vi "Caraya Test for Find Complete Frame.vi"() -> ()   [LabVIEW 2018]
uses:
  Libraries/iTacho_class/iTacho.lvclass
  <vilib>/addons/_JKI Toolkits/Caraya/classes/Test/Test.lvclass
  <vilib>/addons/_JKI Toolkits/Caraya/classes/Assert/Assert.lvclass
panel:
  out "error out":errorcluster
  out "Test Pass?":bool
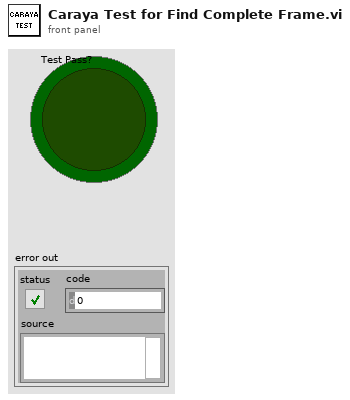
[diagram p1: front panel]
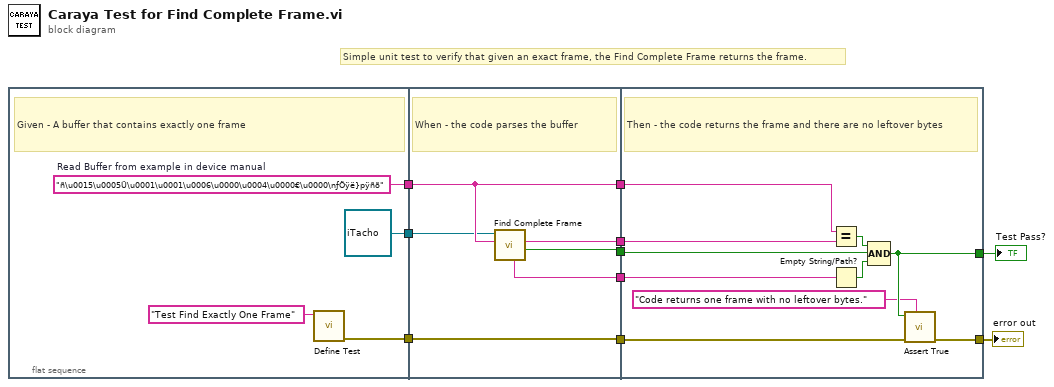
[diagram p0: block diagram]
diagram:
  # "Simple unit test to verify that given an exact frame, the Find Complete Frame returns the frame."
  n1 = flat-sequence {
    tunnel: [refnum<class "iTacho.lvclass"> refnum ("iTacho in")] -> w10
    tunnel: [w13] -> w9
    tunnel: [w11] -> w2
    tunnel: w10 -> [w19]
    tunnel: w9 -> [w20]
    tunnel: [w20] -> w8
    tunnel: [w18] -> w7
    tunnel: [w17] -> w6
    tunnel: [w16] -> w5
    tunnel: [w15] -> w3
    tunnel: w2 -> [w15]
    tunnel: w8 -> [w25]
    tunnel: w7 -> [w28]
    tunnel: w6 -> [w26]
    tunnel: w5 -> [w27]
    tunnel: [w23] -> w4
    tunnel: w3 -> [w24]
    tunnel: [w21] -> w1
    frame #0 {
      w13 = "ñ\u0015\u0005Ü\u0001\u0001\u0006\u0000\u0004\u0000€\u0000\nƒÖÿë}pÿñõ"  # Read Buffer from example in device manual
      # "Given - A buffer that contains exactly one frame"
      n2 = call <vilib>:"Define Test.vi"("Label (VI Title)"="Test Find Exactly One Frame") -> ("error out"=w11:errorcluster)  [unwired: 10 in]
    }
    frame #1 {
      # "When - the code parses the buffer"
      n3 = call-dynamic "Find Complete Frame.vi"("Read Buffer in"=w20, "iTacho in"=w19) -> ("Found New Frame?"=w18:bool, "Frame"=w17:string, "Leftover Bytes"=w16:string)  [unwired: 5 in, 2 out]
    }
    frame #2 {
      # "Then - the code returns the frame and there are no leftover bytes"
      n4 = Equal?(x=w25, y=w26) -> (x = y?=w29:bool)
      n5 = Empty String/Path?(string/path=w27) -> (empty?=w30:bool)
      n6 = Compound Arithmetic op=AND(w29, w28, w30) -> (w23:bool)
      n7 = call <vilib>:"Assert True.vi"("Label"="Code returns one frame with no leftover bytes.", "error in (no error)"=w24, "True?"=w23) -> ("error out"=w21:errorcluster)  [unwired: 8 in]
    }
  }
  "Test Pass?" <- w4
  "error out" <- w1
